vi "MODE_SET_format.vi"(11 "MOTOR_PARAM":T1={"DRIVER_MODE"=enum."CURRENT", "MOTOR_Type_42"=enum."FL57STH41-2804 1.8 deg", "MICROSTEPPING"=enum."1", "WORK_CURRENT"=enum."2.8A", "STOP_CURRENT"=enum."25%"}) -> (3 "Data":u32)   [LabVIEW 2021, in "SMSD.lvclass"]
uses:
  SMSD.lvclass
  Data Unit/SMSD Data Unit/MOTOR_PARAM.ctl
  Data Unit/SMSD Data Unit/DRIVER_MODE.ctl
  Data Unit/SMSD Data Unit/MOTOR_Type_42.ctl
  Data Unit/SMSD Data Unit/MICROSTEPPING.ctl
  Data Unit/SMSD Data Unit/WORK_CURRENT.ctl
  Data Unit/SMSD Data Unit/STOP_CURRENT.ctl
  Data Unit/SMSD Data Unit/SMSD Data Unit.lvclass
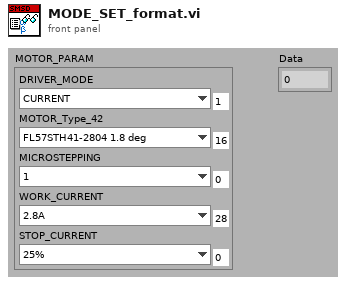
[diagram p1: front panel]
types:
  T1 = typedef "SMSD Data Unit.lvclass/MOTOR_PARAM.ctl" = cluster{"DRIVER_MODE":T2, "MOTOR_Type_42":T3, "MICROSTEPPING":T4, "WORK_CURRENT":T5, "STOP_CURRENT":T6}
  T2 = typedef "SMSD Data Unit.lvclass/DRIVER_MODE.ctl" = enum16{"VOLTAGE", "CURRENT"}
  T3 = typedef "SMSD Data Unit.lvclass/MOTOR_Type_42.ctl" = enum16{"Unknown", "FL42STH33-1334 1.8 deg", "FL42STH33-1334 0.9 deg", "FL42STH38-1206 0.9 deg", "FL42STH38-1684 1.8 deg", "FL42STH38-1684 0.9 deg", "FL42STH47-1206 1.8 deg", "FL42STH47-1684 1.8 deg", "FL42STH47-1684 0.9 deg", "FL42STH60-1206 1.8 deg", "FL42STH60-1206 0.9 deg", "FL57ST41-1564 1.8 deg", "FL57ST76-1006 1.8 deg", "FL57ST76-1506 1.8 deg", "FL57STH41-1006 1.8 deg", "FL57STH41-1006 0.9 deg", "FL57STH41-2804 1.8 deg", "FL57STH41-2804 0.9 deg", "FL57STH51-1006 1.8 deg", "FL57STH51-2804 1.8 deg", "FL57STH51-2804 0.9 deg", "FL57STH56-1006 1.8 deg", "FL57STH56-2006 1.8 deg", "FL57STH56-2804 1.8 deg", "FL57STH76-1006 1.8 deg", "FL57STH76-2804 1.8 deg", "FL57STH76-2804 0.9 deg", "FL60STH65-2008 1.8 deg parallel", "FL60STH65-2008 1.8 deg serial", "FL60STH86-2008 1.8 deg parallel", "FL60STH86-2008 1.8 deg serial", "FL86STH65-2808 1.8 deg parallel", "FL86STH65-2808 1.8 deg serial", "FL86STH80-4208 1.8 deg parallel", "FL86STH80-4208 1.8 deg serial", "FL86STH118-4208 1.8 deg parallel", "FL86STH118-4208 1.8 deg serial", "FL86STH156-4208 1.8 deg parallel", "FL86STH156-4208 1.8 deg serial", "ДШ3934-0,3А", "ДШ2851-0,7А", "ДШ4248-1,7A", "ДШ5776-3,0А", "ДШ57112-3,0А", "ДШ8665-3,0А", "ДШ8682-4,5А"}
  T4 = typedef "SMSD Data Unit.lvclass/MICROSTEPPING.ctl" = enum16{"1", "1/2", "1/4", "1/8", "1/16", "1/32", "1/64", "1/128"}
  T5 = typedef "SMSD Data Unit.lvclass/WORK_CURRENT.ctl" = enum16{"0.0A", "0.1A", "0.2A", "0.3A", "0.4A", "0.5A", "0.6A", "0.7A", "0.8A", "0.9A", "1.0A", "1.1A", "1.2A", "1.3A", "1.4A", "1.5A", "1.6A", "1.7A", "1.8A", "1.9A", "2.0A", "2.1A", "2.2A", "2.3A", "2.4A", "2.5A", "2.6A", "2.7A", "2.8A", "2.9A", "3.0A", "3.1A", "3.2A", "3.3A", "3.4A", "3.5A", "3.6A", "3.7A", "3.8A", "3.9A", "4.0A", "4.1A", "4.2A", "4.3A", "4.4A", "4.5A", "4.6A", "4.7A", "4.8A", "4.9A", "5.0A", "5.1A", "5.2A", "5.3A", "5.4A", "5.5A", "5.6A", "5.7A", "5.8A", "5.9A", "6.0A", "6.1A", "6.2A", "6.3A", "6.4A", "6.5A", "6.6A", "6.7A", "6.8A", "6.9A", "7.0A", "7.1A", "7.2A", "7.3A", "7.4A", "7.5A", "7.6A", "7.7A", "7.8A", "7.9A", "8.0A", "8.1A", "8.2A"}
  T6 = typedef "SMSD Data Unit.lvclass/STOP_CURRENT.ctl" = enum16{"25%", "50%", "75%", "100%"}
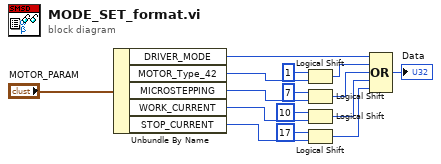
[diagram p0: block diagram]
diagram:
  n1 = Unbundle By Name("MOTOR_PARAM") -> ("DRIVER_MODE"=w6:T2, "MOTOR_Type_42"=w10:T3, "MICROSTEPPING"=w9:T4, "WORK_CURRENT"=w8:T5, "STOP_CURRENT"=w7:T6)
  n2 = Logical Shift(y=i16 1, x=w10) -> (x << y=w5:u32)
  n3 = Logical Shift(y=i16 7, x=w9) -> (x << y=w4:u32)
  n4 = Logical Shift(y=i16 10, x=w8) -> (x << y=w3:u32)
  n5 = Logical Shift(y=i16 17, x=w7) -> (x << y=w2:u32)
  n6 = Compound Arithmetic op=OR(w6, w5, w4, w3, w2) -> (→"Data":u32)
